vi "Find Sub-Index.vi"(10 "OD Subentry":refnum<class "OD Subentry.lvclass">=refnum, 11 "OD Entry in":refnum<class "OD Entry.lvclass">) -> (1 "Found?":bool, 2 "Sub-Index":u16, 3 "OD Entry out":refnum<class "OD Entry.lvclass">)   [LabVIEW 2024]
doc: "Looks for a entry in the subindexs, return the index if found"
uses:
  OD Entry.lvclass/OD Entry.ctl
  OD Entry.lvclass
  OD Subentry/OD Subentry.lvclass
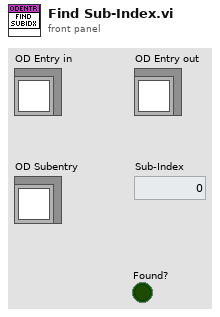
[diagram p1: front panel]
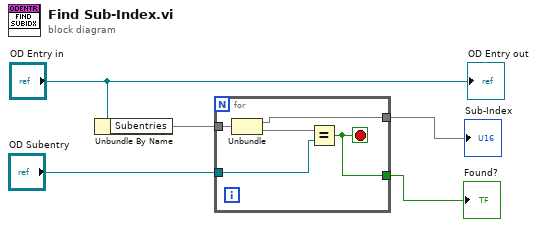
[diagram p0: block diagram]
diagram:
  n1 = Unbundle By Name("OD Entry in") -> ("Subentries"=w4)
  n2 = for {
    tunnel: w4 -> [w10]
    tunnel: "OD Subentry" -> [w8]
    tunnel: [w7] -> w2
    tunnel: [w6] -> w1
    stop <- w6 stop-if-true
    n3 = Unbundle(w10) -> (w7, w9)
    n4 = Equal?(x=w9, y=w8) -> (x = y?=w6:bool)
  }
  "Sub-Index" <- w2
  "Found?" <- w1
  "OD Entry out" <- "OD Entry in"
